vi "Selection to String array.vi"(2 "Selection array":u16[](array[ring]) items=["0", "1", "2"], 3 "String input":string[](array[string])) -> (14 "String array":string[](array[string]))   [LabVIEW 2020]
doc: "This VI returns a string array which contains strings according to the selected value of String input.\nExample: For Selection array = (2,0,1) and String input = (A,B,C) the resulting String array is (C,A,B)."
panel:
  # "This vi returns a string array which contains strings according\nto the selected value of String input.\nExample: For Selection array = (2,0,1) and String input = (A,B,C) the \nresulting String array is (C,A,B)."
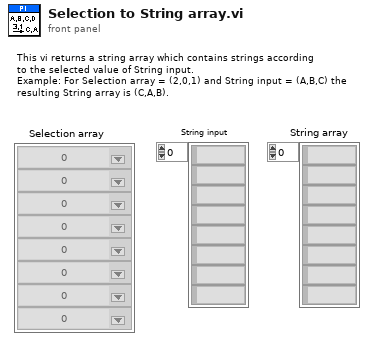
[diagram p1: front panel]
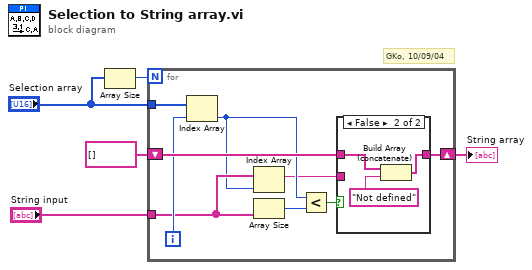
[diagram p0: block diagram]
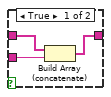
[diagram p2: hidden frame]
diagram:
  # "GKo, 10/09/04"
  n1 = Array Size(array="Selection array") -> (size(s)=w5:i32)
  n2 = for {
    N: w5 -> [_]
    shift-right: [w14] -> w1
    shift-left: string[] [] -> [w13]
    tunnel: "String input" -> [w10]
    tunnel: "Selection array" -> [w12]
    i -> [w11]
    n3 = Index Array(array=w12, index=w11) -> (element=w7:u16)
    n4 = Index Array(array=w10, index=w7) -> (element=w6:string)
    n5 = Array Size(array=w10) -> (size(s)=w9:i32)
    n6 = Less?(x=w7, y=w9) -> (x < y?=w8:bool)
    n7 = case shown="False" w8 {
      tunnel: [w17 w20] -> w14
      tunnel: w13 -> [w16 w19]
      tunnel: w6 -> [w15 _]
      frame True {
        n8 = Build Array (concatenate)(w16, w15) -> (w17:string[])
      }
      frame False {
        n9 = Build Array (concatenate)(w19, "Not defined" ("Input Element")) -> (w20:string[])
      }
    }
  }
  "String array" <- w1
